vi "TCP READ DBL.vi"(8 "error In":errorcluster, 9 "Length":i32=100, 10 "Start Address":i32=1350, 11 "connection ID IN":refnum<k5>) -> (0 "error out":errorcluster, 1 "BArcode":string, 2 "Data":dbl[](array[numeric]) format="%#.6f", 3 "connection ID OUT":refnum<k5>, 5 "Array 2":string[](array[string]), 7 "substring 3":string)   [LabVIEW 2015]
panel:
  out "Array":string[](array[string])
  out "concatenated string":string
  out "substring 2":string
  out "bytes written1":i32
  # "00325"
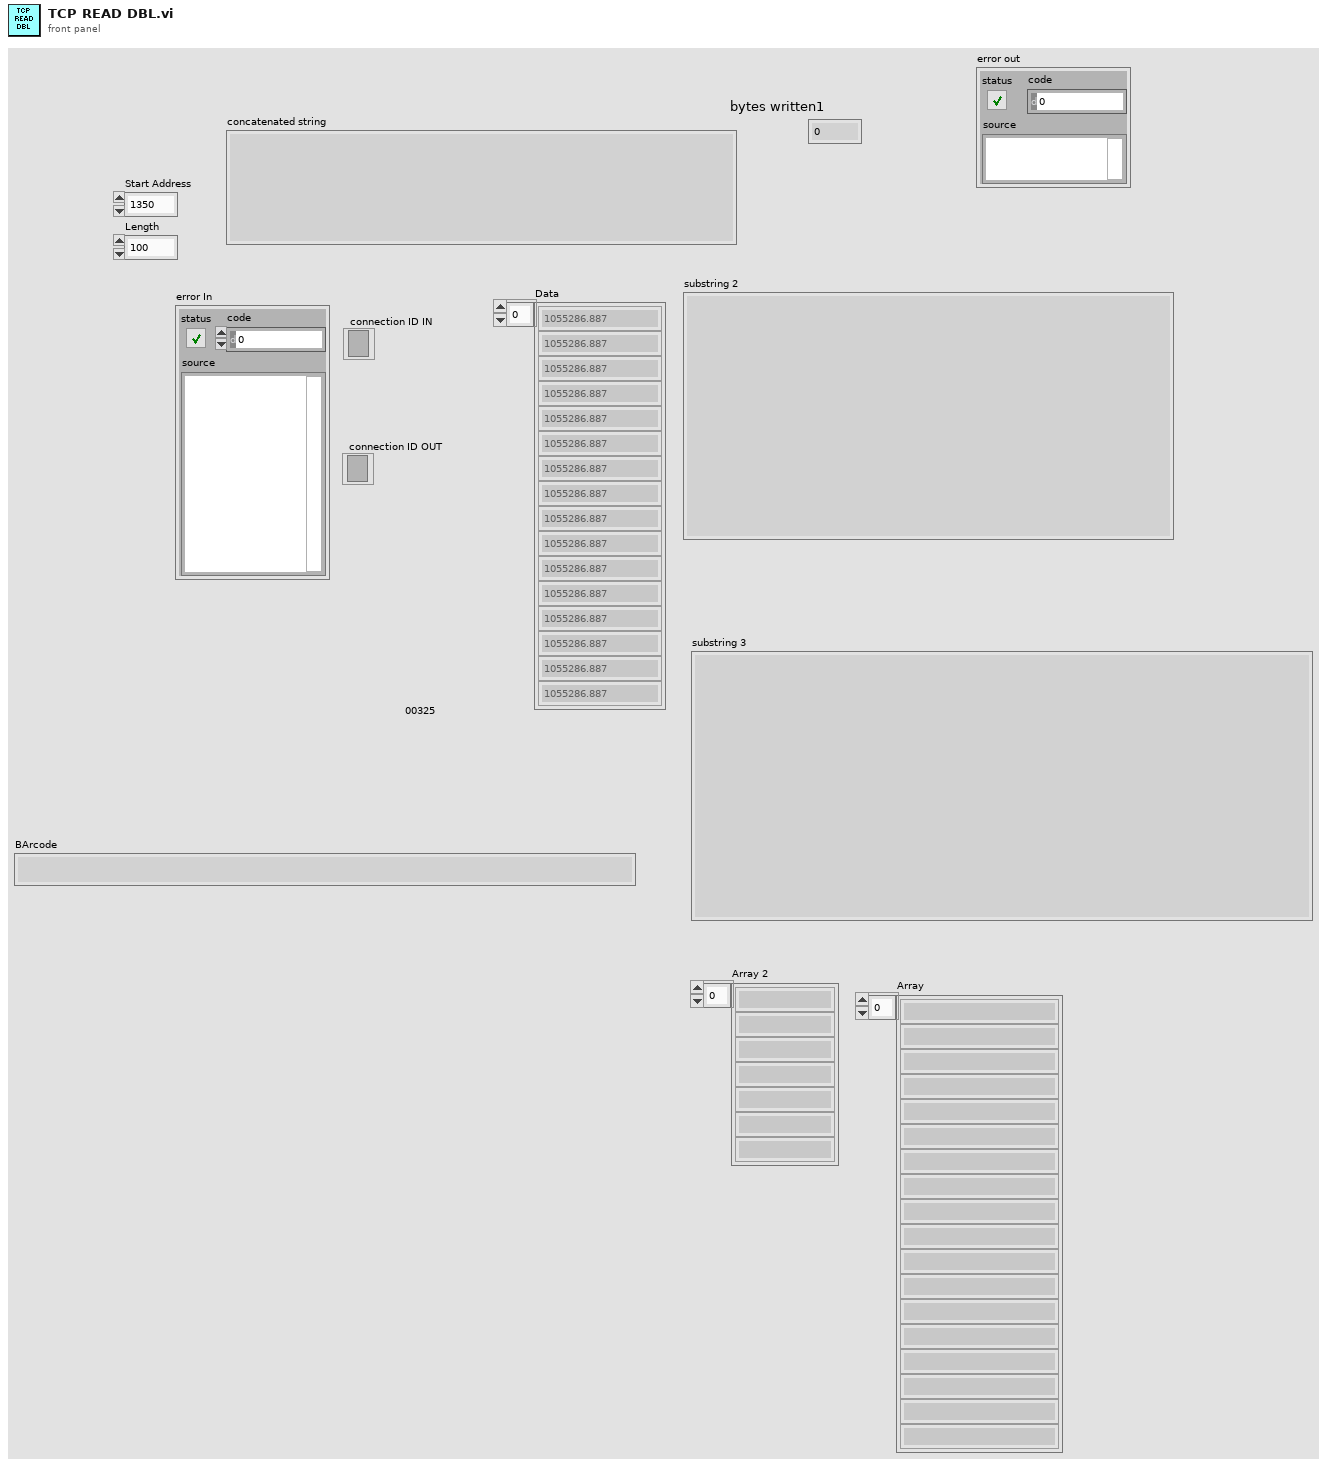
[diagram p1: front panel]
types:
  T1 = enum16{"Standard", "Buffered", "CRLF", "Immediate"}
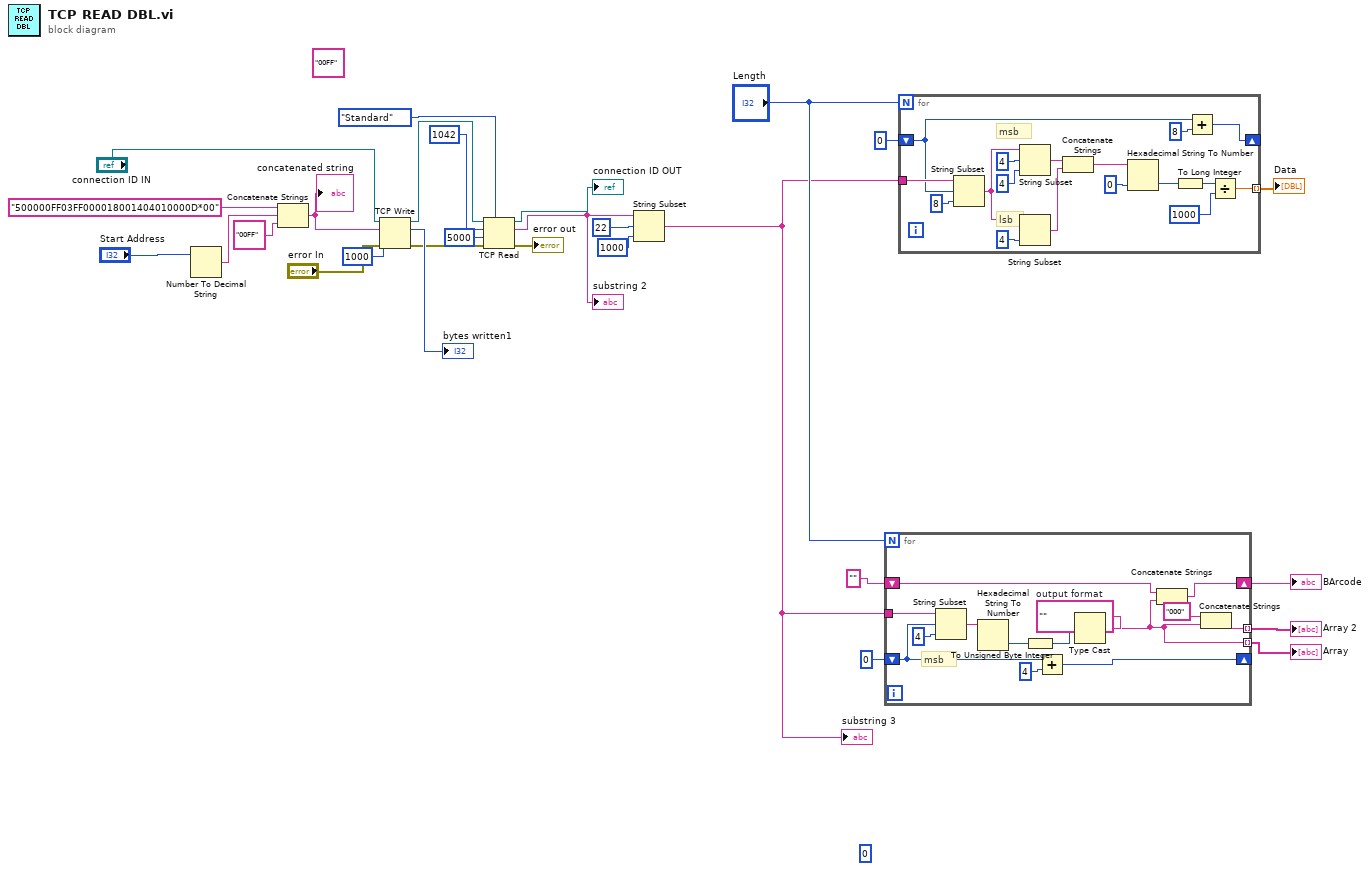
[diagram p0: block diagram]
diagram:
  (unwired) 0
  (unwired) "00FF" ("String")
  n1 = Number To Decimal String(number="Start Address") -> (decimal integer string=w25:string)  [unwired: 1 in]
  n2 = Concatenate Strings("500000FF03FF000018001404010000D*00", w25, "00FF" ("String")) -> (w27:string)
  "concatenated string" <- w27
  n3 = TCP Write(connection ID="connection ID IN", data in=w27, error in (no error)="error In", 9:1000 ("timeout ms (25000)")) -> (connection ID out=w20:refnum<k5>, bytes written=→"bytes written1":i32, error out=w18:errorcluster)
  n4 = TCP Read(connection ID=w20, bytes to read=1042, error in (no error)=w18, 7:T1."Standard" ("mode (standard)"), 9:5000 ("timeout ms (25000)")) -> (connection ID out=→"connection ID OUT":refnum<k5>, data out=w16:string, error out=→"error out":errorcluster)
  "substring 2" <- w16
  n5 = String Subset(string=w16, offset (0)=22, length (rest)=1000 ("length (rest)")) -> (substring=w4:string)
  "substring 3" <- w4
  n6 = for {
    N: "Length" -> [_]
    shift-right: [w42] -> _
    shift-left: 0 -> [w38]
    tunnel: w4 -> [w39]
    tunnel: [w31] -> w8 mode=indexing
    shift-right: [w32] -> w6
    shift-left: "" -> [w33]
    tunnel: [w29] -> w3 mode=indexing
    w35 = ""  # output format
    # "msb"
    n7 = String Subset(string=w39, offset (0)=w38, length (rest)=4 ("length (rest)")) -> (substring=w34:string)
    n8 = Hexadecimal String To Number(string=w34) -> (number=w37:u32)  [unwired: 2 in, 1 out]
    n9 = To Unsigned Byte Integer(number=w37) -> (unsigned 8bit integer=w36:u8)
    n10 = Add(x=w38, y=4) -> (x+y=w42:i32)
    n11 = Type Cast(type=w35, x=w36) -> (*(type *) &x=w29:string)
    n12 = Concatenate Strings(w33, w29) -> (w32:string)
    n13 = Concatenate Strings("000" ("string"), w29) -> (w31:string)
  }
  "Array 2" <- w8
  "BArcode" <- w6
  "Array" <- w3
  n14 = for {
    N: "Length" -> [_]
    shift-right: [w59] -> _
    shift-left: 0 -> [w56]
    tunnel: w4 -> [w57]
    tunnel: [w43] -> w10 mode=indexing
    # "lsb"
    # "msb"
    n15 = String Subset(string=w57, offset (0)=w56, length (rest)=8 ("length (rest)")) -> (substring=w51:string)
    n16 = String Subset(string=w51, offset (0)=4, length (rest)=4 ("length (rest)")) -> (substring=w50:string)
    n17 = String Subset(string=w51, length (rest)=4 ("length (rest)")) -> (substring=w49:string)  [unwired: 1 in]
    n18 = Concatenate Strings(w50, w49) -> (w48:string)
    n19 = Hexadecimal String To Number(string=w48, default (0uL)=u32 0 ("default (0 U32)")) -> (number=w44:u32)  [unwired: 1 in, 1 out]
    n20 = To Long Integer(number=w44) -> (32bit integer=w45:i32)
    n21 = Add(x=w56, y=8) -> (x+y=w59:i32)
    n22 = Divide(x=w45, y=u32 1000) -> (x/y=w43:dbl)
  }
  "Data" <- w10
